vi "Design Challenge.vi"() -> ()   [LabVIEW 2019]
panel:
  in  "?":bool
  in  "?":bool
  out "Trajectory":cluster{"X":dbl, "Y":dbl}[](graph)
  in  "Angle":dbl
  in  "Ho":dbl
  in  "Vo":dbl
  in  "Mass":dbl
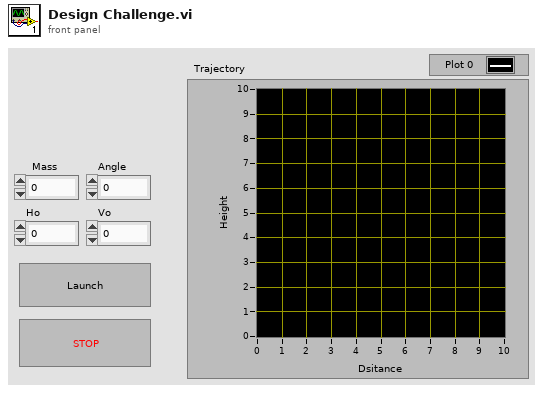
[diagram p1: front panel]
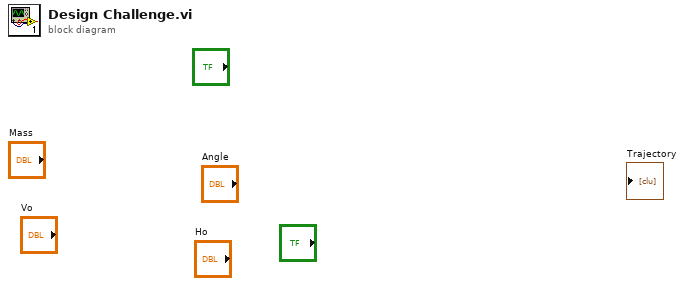
[diagram p0: block diagram]
diagram:
